vi "Shooters and Transfer.vi"(8 "Time":dbl, 9 "Transfer Speed":dbl) -> ()   [LabVIEW 2015]
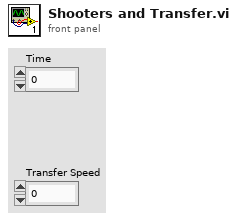
[diagram p1: front panel]
types:
  T1 = typedef "WPI_MotorControlDeviceRef.ctl" = cluster{"DeviceStatus":errorcluster, "Type":T2, "PWM":cluster{"PWM Channel":T3, "DeadBand":T4}, "CAN":cluster{"Device Number":u8, "Control Mode":T5, "Semaphore":T6, "Max Vout":dbl, "TalonSRX Control Mode":T7}, "Invert":bool}
  T2 = typedef "WPI_MotorControlType.ctl" = enum16{"PWM", "CAN", "CANTalonSRX"}
  T3 = typedef "FPGA_DIOPWMChannel.ctl" = enum8{"PWM 0", "PWM 1", "PWM 2", "PWM 3", "PWM 4", "PWM 5", "PWM 6", "PWM 7", "PWM 8", "PWM 9", "PWM MXP 0", "PWM MXP 1", "PWM MXP 2", "PWM MXP 3", "PWM MXP 4", "PWM MXP 5", "PWM MXP 6", "PWM MXP 7", "PWM MXP 8", "PWM MXP 9", "Invalid"}
  T4 = typedef "WPI_PWMDeadband.ctl" = cluster{"Name":string, "maxPositivePwm":i32, "minPositivePwm":i32, "centerPwm":i32, "maxNegativePwm":i32, "minNegativePwm":i32, "angularRange":u16}
  T5 = typedef "WPI_CANJaguar_ControlMode.ctl" = enum8{"Percent VBus", "Current", "Speed", "Position", "Voltage"}
  T6 = typedef "Semaphore RefNum" = refnum<k1>
  T7 = typedef "WPI_CANTalonSRX_APIControlMode.ctl" = enum8{"Percent VBus", "Speed", "Position", "Slave", "Unchanged / Invalid", "Voltage Compensation", "Current", "Motion Profile"}
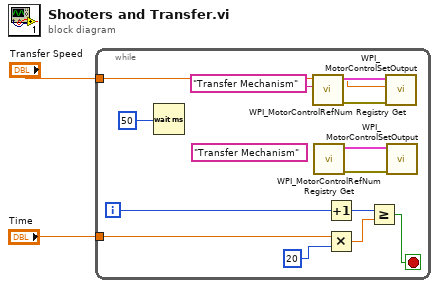
[diagram p0: block diagram]
diagram:
  n1 = while {
    tunnel: "Time" -> [w9]
    tunnel: "Transfer Speed" -> [w6]
    i -> [w8]
    stop <- w7 stop-if-true
    (unwired) "Transfer Mechanism" ("refnum name")
    n2 = Wait (ms)(milliseconds to wait=50) -> ()  [unwired: 1 out]
    n3 = call <vilib>:"WPI_MotorControlRefNum Registry Get.vi"("refnum name"="Transfer Mechanism") -> ("error out"=w16:errorcluster, "MotorControlDevRef"=w14:T1)  [unwired: 9 in]
    n4 = call <vilib>:"WPI_MotorControlRefNum Registry Get.vi"() -> ("error out"=w3:errorcluster, "MotorControlDevRef"=w4:T1)  [unwired: 10 in]
    n5 = Increment(x=w8) -> (x+1=w12:i32)
    n6 = Multiply(x=w9, y=20) -> (x*y=w11:dbl)
    n7 = Greater Or Equal?(x=w12, y=w11) -> (x >= y?=w7:bool)
    n8 = call <vilib>:"WPI_MotorControlSetOutput.vi"("error in (no error)"=w16, "Output"=w6, "MotorControlDevRef"=w14) -> ()  [unwired: 6 in, 3 out]
    n9 = call <vilib>:"WPI_MotorControlSetOutput.vi"("error in (no error)"=w3, "MotorControlDevRef"=w4) -> ("Output"=w5:dbl)  [unwired: 6 in, 3 out]
  }
